vi "日期字符串转时间格式.vi"(11 "data[0]":string) -> (3 "time stamp":timestamp format="%<%Y/%m/%d %H:%M:%S>T")   [LabVIEW 2016, in "潮位站数据传输.lvlib" / "HJ212.lvclass"]
uses:
  HJ212.lvclass
  <vilib>/Utility/miscctls.llb/LVDateTimeRec.ctl
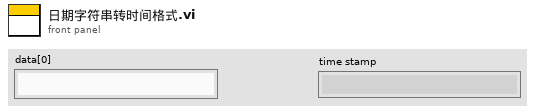
[diagram p1: front panel]
types:
  T1 = typedef "LVDateTimeRec.ctl" = cluster{"fractional second":dbl, "second":i32, "minute":i32, "hour":i32, "day of month":i32, "month":i32, "year":i32, "day of week":i32, "day of year":i32, "DST":i32}
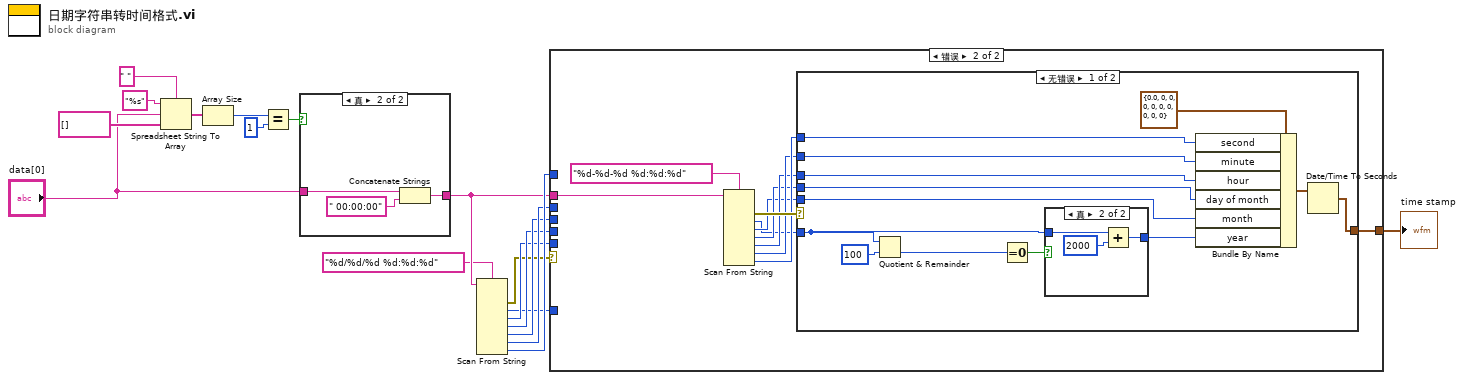
[diagram p0: block diagram]
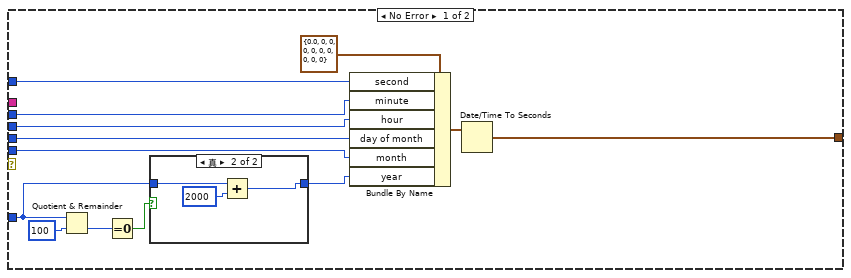
[diagram p3: hidden frame]
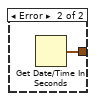
[diagram p6: hidden frame]
diagram:
  n1 = Spreadsheet String To Array(delimiter (Tab)=" " ("分隔符(Tab)"), format string="%s" ("格式字符串"), spreadsheet string="data[0]", array type (2D Dbl)=string[] []) -> (array=w7:string[])
  n2 = Array Size(array=w7) -> (size(s)=w6:i32)
  n3 = Equal?(x=w6, y=1) -> (x = y?=w4:bool)
  n4 = case shown="真" w4 {
    tunnel: "data[0]" -> [w19 w21]
    tunnel: [w19 w20] -> w2
    frame False {
    }
    frame True {
      n5 = Concatenate Strings(w21, " 00:00:00" ("字符串")) -> (w20:string)
    }
  }
  n6 = Scan From String(format string="%d/%d/%d %d:%d:%d" ("格式字符串"), input string=w2) -> (error out=w12:errorcluster, output 1=w13:i32, output 2=w14:i32, output 3=w15:i32, output 4=w16:i32, output 5=w17:i32, output 6=w18:i32)  [unwired: 8 in, 2 out]
  n7 = case shown="错误" w12 {
    tunnel: w18 -> [w34 _]
    tunnel: w17 -> [w33 _]
    tunnel: w16 -> [w32 _]
    tunnel: w15 -> [w31 _]
    tunnel: w14 -> [w30 _]
    tunnel: w13 -> [w26 _]
    tunnel: [w28 w46] -> w11
    tunnel: w2 -> [_ w49]
    frame No Error {
      n8 = Quotient & Remainder(x=w26, y=100) -> (floor(x/y)=w25:i32)  [unwired: 1 out]
      n9 = Equal To 0?(x=w25) -> (x = 0?=w24:bool)
      n10 = case shown="真" w24 {
        tunnel: w26 -> [w36 w39]
        tunnel: [w36 w37] -> w23
        frame False {
        }
        frame True {
          n11 = Add(x=w39, y=2000) -> (x+y=w37:i32)
        }
      }
      n12 = Bundle By Name(cluster=T1 {"fractional second"=0.0, "second"=0, "minute"=0, "hour"=0, "day of month"=0, "month"=0, "year"=0, "day of week"=0, "day of year"=0, "DST"=0} ("日期时间记录"), "second"=w34, "minute"=w33, "hour"=w32, "day of month"=w31, "month"=w30, "year"=w23) -> (w35:T1)
      n13 = Date/Time To Seconds(2:w35) -> (0:w28:timestamp)  [unwired: 1 in]
    }
    frame Error {
      n14 = Scan From String(format string="%d-%d-%d %d:%d:%d" ("格式字符串"), input string=w49) -> (error out=w47:errorcluster, output 1=w40:i32, output 2=w41:i32, output 3=w42:i32, output 4=w43:i32, output 5=w44:i32, output 6=w45:i32)  [unwired: 8 in, 2 out]
      n15 = case shown="无错误" w47 {
        tunnel: [w56 w67] -> w46
        tunnel: w45 -> [w55 _]
        tunnel: w44 -> [w54 _]
        tunnel: w43 -> [w53 _]
        tunnel: w42 -> [w52 _]
        tunnel: w41 -> [w51 _]
        tunnel: w40 -> [w50 _]
        frame No Error {
          n16 = Quotient & Remainder(x=w50, y=100) -> (floor(x/y)=w59:i32)  [unwired: 1 out]
          n17 = Equal To 0?(x=w59) -> (x = 0?=w58:bool)
          n18 = case shown="真" w58 {
            tunnel: w50 -> [w63 w66]
            tunnel: [w63 w64] -> w57
            frame False {
            }
            frame True {
              n19 = Add(x=w66, y=2000) -> (x+y=w64:i32)
            }
          }
          n20 = Bundle By Name(cluster=T1 {"fractional second"=0.0, "second"=0, "minute"=0, "hour"=0, "day of month"=0, "month"=0, "year"=0, "day of week"=0, "day of year"=0, "DST"=0} ("日期时间记录"), "second"=w55, "minute"=w54, "hour"=w53, "day of month"=w52, "month"=w51, "year"=w57) -> (w62:T1)
          n21 = Date/Time To Seconds(2:w62) -> (0:w56:timestamp)  [unwired: 1 in]
        }
        frame Error {
          n22 = Get Date/Time In Seconds() -> (seconds since 1Jan1904=w67:timestamp)
        }
      }
    }
  }
  "time stamp" <- w11
